vi "ExecuteCommand.vi"(10 "Params":string[][](array[string]), 11 "Command":string) -> ()   [LabVIEW 2018]
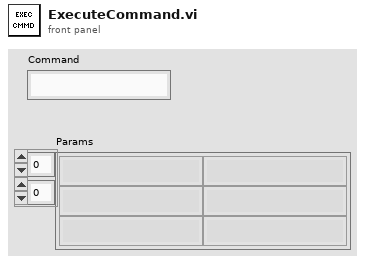
[diagram p1: front panel]
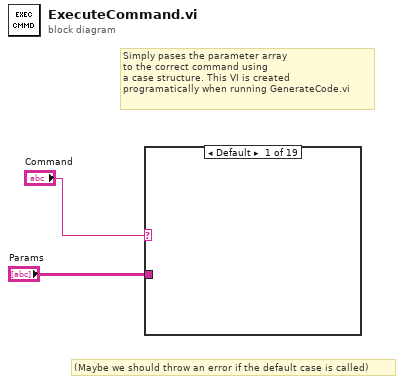
[diagram p0: block diagram]
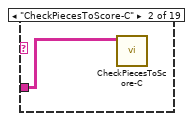
[diagram p2: hidden frame]
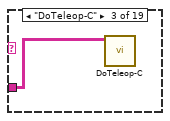
[diagram p3: hidden frame]
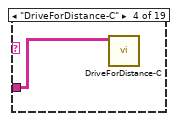
[diagram p4: hidden frame]
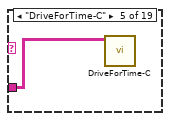
[diagram p5: hidden frame]
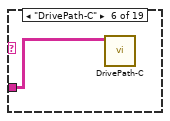
[diagram p6: hidden frame]
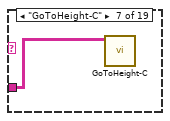
[diagram p7: hidden frame]
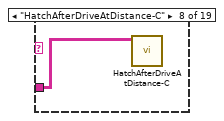
[diagram p8: hidden frame]
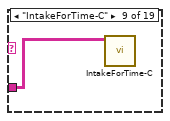
[diagram p9: hidden frame]
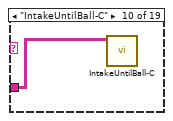
[diagram p10: hidden frame]
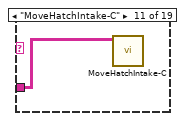
[diagram p11: hidden frame]
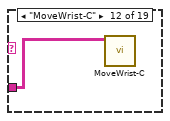
[diagram p12: hidden frame]
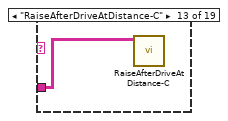
[diagram p13: hidden frame]
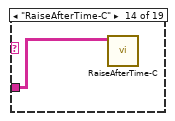
[diagram p14: hidden frame]
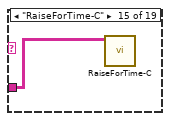
[diagram p15: hidden frame]
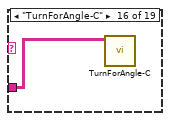
[diagram p16: hidden frame]
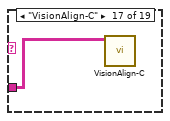
[diagram p17: hidden frame]
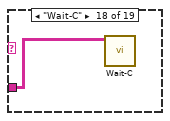
[diagram p18: hidden frame]
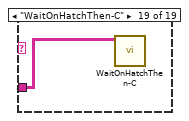
[diagram p19: hidden frame]
diagram:
  # "(Maybe we should throw an error if the default case is called)"
  # "Simply pases the parameter array\nto the correct command using\na case structure. This VI is created\nprogramatically when running GenerateCode.vi"
  n1 = case shown="Default" "Command" {
    tunnel: "Params" -> [_ w3 w4 w5 w6 w7 w8 w9 w10 w11 w12 w13 w14 w15 w16 w17 w18 w19 w20]
    frame Default {
    }
    frame "CheckPiecesToScore-C" {
      n2 = call "CheckPiecesToScore-C.vi"("Params"=w3) -> ()  [unwired: 11 in]
    }
    frame "DoTeleop-C" {
      n3 = call "DoTeleop-C.vi"("Params"=w4) -> ()  [unwired: 11 in]
    }
    frame "DriveForDistance-C" {
      n4 = call "DriveForDistance-C.vi"("Params"=w5) -> ()  [unwired: 11 in]
    }
    frame "DriveForTime-C" {
      n5 = call "DriveForTime-C.vi"("Params"=w6) -> ()  [unwired: 11 in]
    }
    frame "DrivePath-C" {
      n6 = call "DrivePath-C.vi"("Params"=w7) -> ()  [unwired: 11 in]
    }
    frame "GoToHeight-C" {
      n7 = call "GoToHeight-C.vi"("Params"=w8) -> ()  [unwired: 11 in]
    }
    frame "HatchAfterDriveAtDistance-C" {
      n8 = call "HatchAfterDriveAtDistance-C.vi"("Params"=w9) -> ()  [unwired: 11 in]
    }
    frame "IntakeForTime-C" {
      n9 = call "IntakeForTime-C.vi"("Params"=w10) -> ()  [unwired: 11 in]
    }
    frame "IntakeUntilBall-C" {
      n10 = call "IntakeUntilBall-C.vi"("Params"=w11) -> ()  [unwired: 11 in]
    }
    frame "MoveHatchIntake-C" {
      n11 = call "MoveHatchIntake-C.vi"("Params"=w12) -> ()  [unwired: 11 in]
    }
    frame "MoveWrist-C" {
      n12 = call "MoveWrist-C.vi"("Params"=w13) -> ()  [unwired: 11 in]
    }
    frame "RaiseAfterDriveAtDistance-C" {
      n13 = call "RaiseAfterDriveAtDistance-C.vi"("Params"=w14) -> ()  [unwired: 11 in]
    }
    frame "RaiseAfterTime-C" {
      n14 = call "RaiseAfterTime-C.vi"("Params"=w15) -> ()  [unwired: 11 in]
    }
    frame "RaiseForTime-C" {
      n15 = call "RaiseForTime-C.vi"("Params"=w16) -> ()  [unwired: 11 in]
    }
    frame "TurnForAngle-C" {
      n16 = call "TurnForAngle-C.vi"("Params"=w17) -> ()  [unwired: 11 in]
    }
    frame "VisionAlign-C" {
      n17 = call "VisionAlign-C.vi"("Params"=w18) -> ()  [unwired: 11 in]
    }
    frame "Wait-C" {
      n18 = call "Wait-C.vi"("Params"=w19) -> ()  [unwired: 11 in]
    }
    frame "WaitOnHatchThen-C" {
      n19 = call "WaitOnHatchThen-C.vi"("Params"=w20) -> ()  [unwired: 11 in]
    }
  }
